vi "clean-expSD.vi"(1 "Update graphs of exp":refnum<user-event>, 2 "input cluster":T1={"Kinetics"=[], "Spectrum"=[], "Experiments groups"=[], "GRAPH EXPERIMENTAL DATA"=[], "error out"={"status"=FALSE, "code"=0, "source"=""}, "group"=0, "exp selected"=0, "# exp"=0, "kinetics plot names"=[], "spectra plot names"=[], "FromToWave"={"FromWave"=0.0, "ToWave"=0.0}, "Laser shutter task"="", "Accelerator task"="", "Motor task"="", "GRAPH EXPERIMENTAL DATA ref"=refnum, "timedelays"=[0.0, 0.0, 0.0, 0.0, 0.0, 0.0, 0.0, 0.06019061100911815, 0.0521779104562645, 0.045231877429679615, 0.03921051490799832, 0.033990728811568754, 0.029465811603150715, 0.025543260876973825, 0.02214288834180205, 0.01919518054014414, 0.016639877791965713, 0.014424742312398925, 0.012504490320209958, 0.010839866306230088, 0.009396840537117498, 0.008145913389103785, 0.00706151229029317, 0.006121468943269439, 0.005306566140927374, 0.004600144911132549, 0.003987763959109073, 0.0034569044455719407, 0.00299671406541447, 0.0025977851951783253, 0.0022519625739982996, 0.00195217658646366, 0.0016922987392150965, 0.0014670163768006634, 0.0012717240756200802, 0.0011024294957352762, 0.0009556717658856477, 0.0008284507332614981, 0.0007181656316962257, 0.0006225619144775864, 0.0005396851648867825, 0.00046784114226338394, 0.0004055611468220084, 0.0003515719951773376, 0.00030476999279031153, 0.00026419837125694315, 0.00022902772919263772, 0.0001985390768670671, 0.0001721091379728629, 0.00014919760805372974, 0.00012933610911736794], "wavelengths"=[0.0, 0.0, 0.0, 0.0, 0.0, 0.0, 0.0, 0.06019061100911815, 0.0521779104562645, 0.045231877429679615, 0.03921051490799832, 0.033990728811568754, 0.029465811603150715, 0.025543260876973825, 0.02214288834180205, 0.01919518054014414, 0.016639877791965713, 0.014424742312398925, 0.012504490320209958, 0.010839866306230088, 0.009396840537117498, 0.008145913389103785, 0.00706151229029317, 0.006121468943269439, 0.005306566140927374, 0.004600144911132549, 0.003987763959109073, 0.0034569044455719407, 0.00299671406541447, 0.0025977851951783253, 0.0022519625739982996, 0.00195217658646366, 0.0016922987392150965, 0.0014670163768006634, 0.0012717240756200802, 0.0011024294957352762, 0.0009556717658856477, 0.0008284507332614981, 0.0007181656316962257, 0.0006225619144775864, 0.0005396851648867825, 0.00046784114226338394, 0.0004055611468220084, 0.0003515719951773376, 0.00030476999279031153, 0.00026419837125694315, 0.00022902772919263772, 0.0001985390768670671, 0.0001721091379728629, 0.00014919760805372974, 0.00012933610911736794], "Experiment"=refnum, "Commentaires exp"=refnum, "FromToDelay"={"FromDelay"=0.0, "ToDelay"=0.0}}) -> (0 "output cluster":T1={"Kinetics"=[], "Spectrum"=[], "Experiments groups"=[], "GRAPH EXPERIMENTAL DATA"=[], "error out"={"status"=FALSE, "code"=0, "source"=""}, "group"=0, "exp selected"=0, "# exp"=0, "kinetics plot names"=[], "spectra plot names"=[], "FromToWave"={"FromWave"=0.0, "ToWave"=0.0}, "Laser shutter task"="", "Accelerator task"="", "Motor task"="", "GRAPH EXPERIMENTAL DATA ref"=refnum, "timedelays"=[0.0, 0.0, 0.0, 0.0, 0.0, 0.0, 0.0, 0.06019061100911815, 0.0521779104562645, 0.045231877429679615, 0.03921051490799832, 0.033990728811568754, 0.029465811603150715, 0.025543260876973825, 0.02214288834180205, 0.01919518054014414, 0.016639877791965713, 0.014424742312398925, 0.012504490320209958, 0.010839866306230088, 0.009396840537117498, 0.008145913389103785, 0.00706151229029317, 0.006121468943269439, 0.005306566140927374, 0.004600144911132549, 0.003987763959109073, 0.0034569044455719407, 0.00299671406541447, 0.0025977851951783253, 0.0022519625739982996, 0.00195217658646366, 0.0016922987392150965, 0.0014670163768006634, 0.0012717240756200802, 0.0011024294957352762, 0.0009556717658856477, 0.0008284507332614981, 0.0007181656316962257, 0.0006225619144775864, 0.0005396851648867825, 0.00046784114226338394, 0.0004055611468220084, 0.0003515719951773376, 0.00030476999279031153, 0.00026419837125694315, 0.00022902772919263772, 0.0001985390768670671, 0.0001721091379728629, 0.00014919760805372974, 0.00012933610911736794], "wavelengths"=[0.0, 0.0, 0.0, 0.0, 0.0, 0.0, 0.0, 0.06019061100911815, 0.0521779104562645, 0.045231877429679615, 0.03921051490799832, 0.033990728811568754, 0.029465811603150715, 0.025543260876973825, 0.02214288834180205, 0.01919518054014414, 0.016639877791965713, 0.014424742312398925, 0.012504490320209958, 0.010839866306230088, 0.009396840537117498, 0.008145913389103785, 0.00706151229029317, 0.006121468943269439, 0.005306566140927374, 0.004600144911132549, 0.003987763959109073, 0.0034569044455719407, 0.00299671406541447, 0.0025977851951783253, 0.0022519625739982996, 0.00195217658646366, 0.0016922987392150965, 0.0014670163768006634, 0.0012717240756200802, 0.0011024294957352762, 0.0009556717658856477, 0.0008284507332614981, 0.0007181656316962257, 0.0006225619144775864, 0.0005396851648867825, 0.00046784114226338394, 0.0004055611468220084, 0.0003515719951773376, 0.00030476999279031153, 0.00026419837125694315, 0.00022902772919263772, 0.0001985390768670671, 0.0001721091379728629, 0.00014919760805372974, 0.00012933610911736794], "Experiment"=refnum, "Commentaires exp"=refnum, "FromToDelay"={"FromDelay"=0.0, "ToDelay"=0.0}})   [LabVIEW 2015]
uses:
  controls/control-cluster.ctl
  Classes/Experiments_group.lvclass
  Classes/Experiment.lvclass
types:
  T1 = typedef "control-cluster.ctl" = cluster{"Kinetics":cluster{"timedelay":dbl[], dbl[]}[], "Spectrum":cluster{"Unités abscisse":dbl[], dbl[]}[], "Experiments groups":refnum<class "Experiments_group.lvclass">[], "GRAPH EXPERIMENTAL DATA":dbl[][], "error out":errorcluster, "group":i32, "exp selected":i32, "# exp":i32, "kinetics plot names":string[], "spectra plot names":string[], "FromToWave":cluster{"FromWave":dbl, "ToWave":dbl}, "Laser shutter task":refnum<k21>, "Accelerator task":refnum<k21>, "Motor task":refnum<k21>, "GRAPH EXPERIMENTAL DATA ref":refnum<vi>, "timedelays":dbl[], "wavelengths":dbl[], "Experiment":refnum<vi>, "Commentaires exp":refnum<vi>, "FromToDelay":cluster{"FromDelay":dbl, "ToDelay":dbl}}
  T2 = cluster{bool, "Item Names":string[], "exp selected":i32}
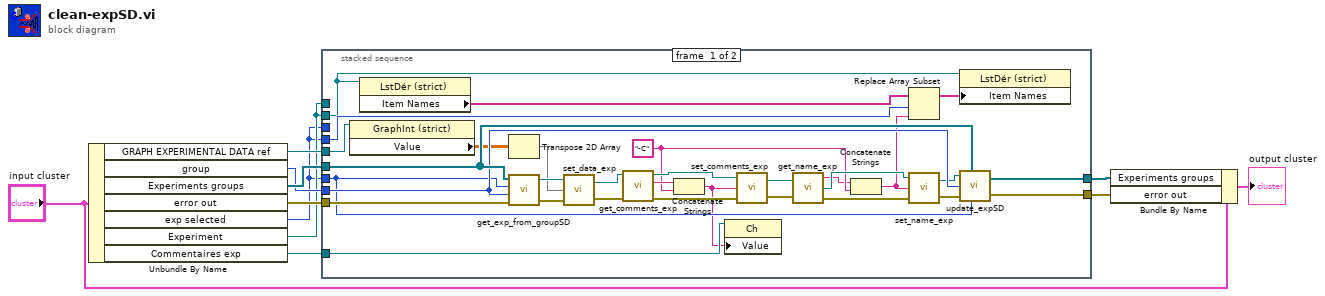
[diagram p0: block diagram]
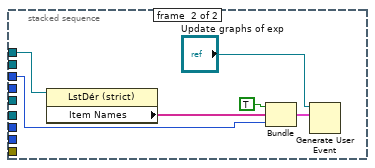
[diagram p2: hidden frame]
diagram:
  n1 = Unbundle By Name("input cluster") -> ("GRAPH EXPERIMENTAL DATA ref"=w11:refnum<vi>, "group"=w6:i32, "Experiments groups"=w7:refnum<class "Experiments_group.lvclass">[], "error out"=w5:errorcluster, "exp selected"=w1:i32, "Experiment"=w2:refnum<vi>, "Commentaires exp"=w3:refnum<vi>)
  n2 = stacked-sequence {
    tunnel: w11 -> [w42 _]
    tunnel: [w41 _] -> w9
    tunnel: [w40 _] -> w8
    tunnel: w7 -> [w39 _]
    tunnel: w6 -> [w38 _]
    tunnel: w5 -> [w37 _]
    tunnel: w1 -> [w32 _]
    tunnel: w1 -> [_ w44]
    tunnel: w2 -> [_ w43]
    tunnel: w3 -> [w26 _]
    tunnel: w2 -> [w13 _]
    tunnel: w1 -> [w15 _]
    frame #0 {
      w21 = "-C" ("chaîne")
      n3 = property class="GraphInt (strict)"(reference=w42) -> ("Value"=w34:dbl[][])  [unwired: 1 in, 2 out]
      n4 = property on="Property Node" class="LstDér (strict)"(reference=w13) -> ("Item Names"=w16:string[])  [unwired: 1 in, 2 out]
      n5 = Transpose 2D Array(2D array=w34) -> (transposed array=w33:dbl[][])
      n6 = call "get_exp_from_groupSD.vi"("error in (no error)"=w37, "group"=w38, "exp selected"=w32, "Experiments groups"=w39) -> ("error out"=w35:errorcluster, "Experiment out"=w36:refnum<class "Experiment.lvclass">)  [unwired: 1 out]
      n7 = call-dynamic "set_data_exp.vi"("error in (no error)"=w35, "Data"=w33, "Experiment.lvclass in"=w36) -> ("error out"=w27:errorcluster, "Experiment.lvclass out"=w31:refnum<class "Experiment.lvclass">)
      n8 = call-dynamic "get_comments_exp.vi"("error in (no error)"=w27, "Experiment.lvclass in"=w31) -> ("error out"=w29:errorcluster, "Comments"=w28:string, "Experiment.lvclass out"=w30:refnum<class "Experiment.lvclass">)  [unwired: 7 in]
      n9 = Concatenate Strings(w28, w21) -> (w25:string)
      n10 = property on="Property Node" class="Ch"(reference=w26, "Value"=w25) -> ()  [unwired: 1 in, 2 out]
      n11 = call-dynamic "set_comments_exp.vi"("error in (no error)"=w29, "Comments"=w25, "Experiment.lvclass in"=w30) -> ("error out"=w23:errorcluster, "Experiment.lvclass out"=w24:refnum<class "Experiment.lvclass">)
      n12 = call-dynamic "get_name_exp.vi"("Experiment.lvclass in"=w24, "error in (no error)"=w23) -> ("Exp name"=w20:string, "Experiment.lvclass out"=w22:refnum<class "Experiment.lvclass">, "error out"=w19:errorcluster)
      n13 = Concatenate Strings(w20, w21) -> (w14:string)
      n14 = Replace Array Subset(array=w16, new element=w14, index=w15) -> (w12:string[])
      n15 = call-dynamic "set_name_exp.vi"("error in (no error)"=w19, "Exp name"=w14, "Experiment.lvclass in"=w22) -> ("error out"=w17:errorcluster, "Experiment.lvclass out"=w18:refnum<class "Experiment.lvclass">)
      n16 = property on="Property Node" class="LstDér (strict)"(reference=w13, "Item Names"=w12) -> ()  [unwired: 1 in, 2 out]
      n17 = call "update_expSD.vi"("Experiment in"=w18, "Experiments groups in"=w39, "group"=w38, "error in (no error)"=w17, "exp selected"=w32) -> ("Experiments groups out"=w41:refnum<class "Experiments_group.lvclass">[], "error out"=w40:errorcluster)
    }
    frame #1 {
      n18 = property on="Property Node" class="LstDér (strict)"(reference=w43) -> ("Item Names"=w46:string[])  [unwired: 1 in, 2 out]
      n19 = Bundle(TRUE, "Item Names"=w46, "exp selected"=w44) -> (w48:T2)  [unwired: 1 in]
      n20 = Generate User Event(user event="Update graphs of exp", event data cluster=w48) -> ()  [unwired: 2 in, 2 out]
    }
  }
  n21 = Bundle By Name(cluster="input cluster", "Experiments groups"=w9, "error out"=w8) -> (→"output cluster":T1)
